vi "Update Pin Map.vi"(8 "error in":errorcluster, 11 "Pin Map Path":string) -> (0 "error out":errorcluster, 3 "Pin Map Id Out":string)   [LabVIEW 2023]
doc: "register pinmap to service"
uses:
  <vilib>/MeasurementLink/MeasurementLink Discovery Client/RPC Messages/ni_measurementlink_discovery_v1_ResolveServiceRequest.ctl
  <vilib>/MeasurementLink/MeasurementLink Pin Map Client/RPC Messages/ni_measurementlink_pinmap_v1_UpdatePinMapFromXmlRequest.ctl
  <vilib>/MeasurementLink/MeasurementLink Measurement Server/MeasurementLink Measurement Server.lvlib
  <vilib>/MeasurementLink/MeasurementLink Discovery Client/MeasurementLink Discovery Client.lvlib
  <vilib>/MeasurementLink/MeasurementLink Pin Map Client/MeasurementLink Pin Map Client.lvlib
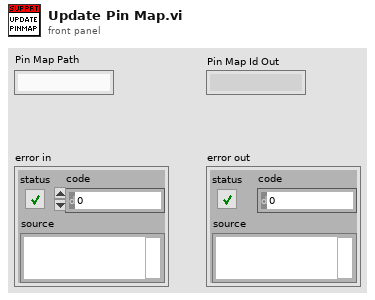
[diagram p1: front panel]
types:
  T1 = typedef "MeasurementLink Pin Map Client.lvlib/ni_measurementlink_pinmap_v1_UpdatePinMapFromXmlRequest.ctl" = cluster{"pin_map_id":string, "pin_map_xml":string}
  T2 = typedef "MeasurementLink Discovery Client.lvlib/ni_measurementlink_discovery_v1_ResolveServiceRequest.ctl" = cluster{"provided_interface":string, "service_class":string}
  T3 = typedef "grpc-lvsupport-release.lvlib/grpcId.ctl" = u64
  T4 = typedef "MeasurementLink Discovery Client.lvlib/ni_measurementlink_discovery_v1_ServiceLocation.ctl" = cluster{"location":string, "insecure_port":string, "ssl_authenticated_port":string}
  T5 = typedef "MeasurementLink Pin Map Client.lvlib/ni_measurementlink_pinmap_v1_PinMap.ctl" = cluster{"pin_map_id":string}
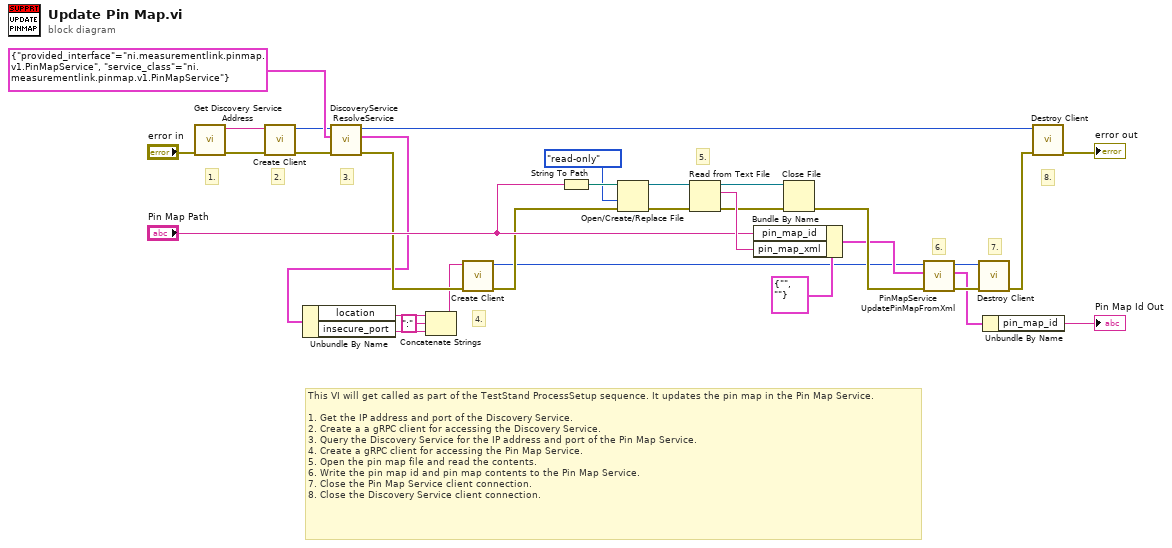
[diagram p0: block diagram]
diagram:
  # "8."
  # "7."
  # "6."
  # "5."
  # "4."
  # "3."
  # "2."
  # "1."
  # "This VI will get called as part of the TestStand ProcessSetup sequence. It updates the pin map in the Pin Map Service. \n\n1. Get the IP address and port of the Discovery Service.\n2. Create a a gRPC client for accessing the Discovery Service.\n3. Query the Discovery Service for the IP address and port of the Pin Map Service.\n4. Create a gRPC client for accessing the Pin Map Service.\n5. Open the pin map file and read the contents.\n6. Write the pin map id and pin map contents to the Pin Map Service.\n7. Close the Pin Map Service client connection.\n8. Close the Discovery Service client connection."
  n1 = call <vilib>:"Get Discovery Service Address.vi"("error in"="error in") -> ("error out"=w32:errorcluster, "address"=w31:string)  [unwired: 9 in]
  n2 = call <vilib>:"Create Client.vi"("error in"=w32, "address"=w31) -> ("error out"=w19:errorcluster, "gRPC ID Out"=w29:T3)  [unwired: 8 in]
  n3 = call <vilib>:"DiscoveryService ResolveService.vi"("error in"=w19, "Request Data"=T2 {"provided_interface"="ni.measurementlink.pinmap.v1.PinMapService", "service_class"="ni.measurementlink.pinmap.v1.PinMapService"}, "gRPC ID"=w29) -> ("error out"=w18:errorcluster, "Response Data"=w2:T4, "gRPC ID out"=w8:T3)  [unwired: 6 in]
  n4 = Unbundle By Name(w2) -> ("location"=w3:string, "insecure_port"=w4:string)
  n5 = Concatenate Strings(w3, ":" ("string"), w4) -> (w1:string)
  n6 = call <vilib>:"Create Client.vi"("error in"=w18, "address"=w1) -> ("error out"=w17:errorcluster, "gRPC ID Out"=w13:T3)  [unwired: 8 in]
  n7 = String To Path(string="Pin Map Path") -> (path=w27:path)
  n8 = Open/Create/Replace File(file path (use dialog)=w27, error in=w17, access (0:read/write)=enum16{"read/write", "read-only", "write-only"}."read-only") -> (refnum out=w24:refnum<file>, error out=w25:errorcluster)  [unwired: 3 in, 1 out]
  n9 = Read from Text File(file (use dialog)=w24, error in=w25) -> (refnum out=w20:refnum<file>, text=w23:string, error out=w21:errorcluster)  [unwired: 2 in, 1 out]
  n10 = Bundle By Name(cluster=T1 {"pin_map_id"="", "pin_map_xml"=""} ("Request Data"), "pin_map_id"="Pin Map Path", "pin_map_xml"=w23) -> (w14:T1)
  n11 = Close File(refnum=w20, error in=w21) -> (error out=w16:errorcluster)  [unwired: 1 out]
  n12 = call <vilib>:"PinMapService UpdatePinMapFromXml.vi"("error in"=w16, "Request Data"=w14, "gRPC ID"=w13) -> ("error out"=w12:errorcluster, "Response Data"=w7:T5, "gRPC ID out"=w11:T3)  [unwired: 6 in]
  n13 = call <vilib>:"Destroy Client.vi"("error in"=w12, "gRPC ID"=w11) -> ("error out"=w10:errorcluster)  [unwired: 9 in]
  n14 = Unbundle By Name(w7) -> ("pin_map_id"=→"Pin Map Id Out":string)
  n15 = call <vilib>:"Destroy Client.vi"("error in"=w10, "gRPC ID"=w8) -> ("error out"=→"error out":errorcluster)  [unwired: 9 in]
